vi "Init with SQL Records.vi"(8 "error in (no error)":errorcluster, 10 "SQL Dataset":variant[][](array[variant]), 11 "Banking Statement in":refnum<class "Banking Statement.lvclass">) -> (0 "error out":errorcluster, 3 "Banking Statement out":refnum<class "Banking Statement.lvclass">)   [LabVIEW 2018, in "Banking Statement.lvclass"]
uses:
  Banking Statement.lvclass
  C:/Users/Jeff Tipps/Documents/Filthy-Lucre-Budgetizer/source/support/classes/Statement/Statement.lvclass
  Banking Record/Banking Transaction.lvclass
  C:/Users/Jeff Tipps/Documents/Filthy-Lucre-Budgetizer/source/support/classes/Transaction/Transaction.lvclass
  Statement/Statement.lvclass/Statement.ctl
  Statement/Statement.lvclass
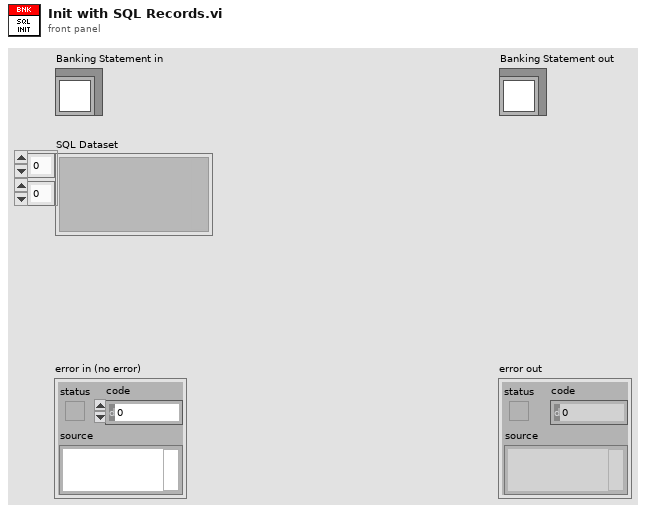
[diagram p1: front panel]
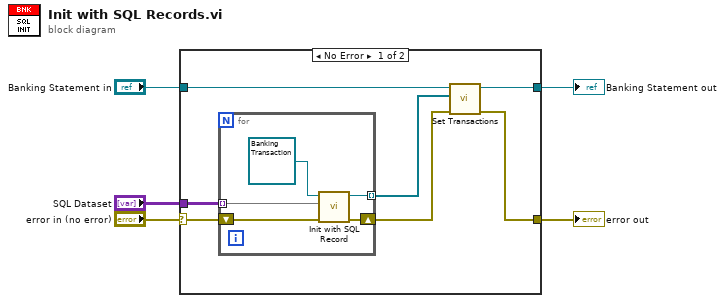
[diagram p0: block diagram]
diagram:
  n1 = case shown="No Error" "error in (no error)" {
    selector: "error in (no error)" -> [w12 w19]
    tunnel: "Banking Statement in" -> [w10 w18]
    tunnel: "SQL Dataset" -> [w11 _]
    tunnel: [w6 w19] -> w4
    tunnel: [w9 w18] -> w5
    frame No Error {
      n2 = for {
        shift-right: [w14] -> w7
        shift-left: w12 -> [w15]
        tunnel: w11 -> [w16] mode=indexing
        tunnel: [w17] -> w8 mode=indexing
        n3 = call-dynamic "Init with SQL Record.vi"("error in (no error)"=w15, "MySQL Record"=w16, "Banking Transaction in"=refnum<class "Banking Transaction.lvclass"> refnum ("Banking Transaction.lvclass")) -> ("error out"=w14:errorcluster, "Banking Transaction out"=w17:refnum<class "Banking Transaction.lvclass">)  [unwired: 7 in]
      }
      n4 = call "Set Transactions.vi"("error in (no error)"=w7, "Transactions"=w8, "Statement in"=w10) -> ("error out"=w6:errorcluster, "Statement out"=w9:refnum<class "Banking Statement.lvclass">)  [unwired: 7 in]
    }
    frame Error {
    }
  }
  "error out" <- w4
  "Banking Statement out" <- w5
